vi "Control - Generic - Smoke Limit Host.vi"() -> ()   [LabVIEW 2015, in "ECS-Host.lvlib"]
uses:
  ECS-Host.lvlib
  <vilib>/addons/Software Calibration Management/XControls/TBL2D.xctl
panel:
  in  "SmokeLimitMode":bool
  in  "_Smoke Limit Mode Tab Control":enum32{"Phi", "Quantity"}(tab)
  in  "SmokeLimitPhi_Tbl":cluster{"X":sgl[], "Y":sgl[], "Z":sgl[][]}(xcontrol)
  out "SmokeLimitPhi_TblOut":sgl caption="[]"
  in  "SmokeLimitFuel_Tbl":cluster{"X":sgl[], "Y":sgl[], "Z":sgl[][]}(xcontrol)
  out "SmokeLimitFuel_TblOut":sgl caption="[mg/cyc]"
  out "FuelLimit_Calc":sgl caption="[]"
  in  "SmokeLimit_E":bool
  out "SmokeLimitActive":bool
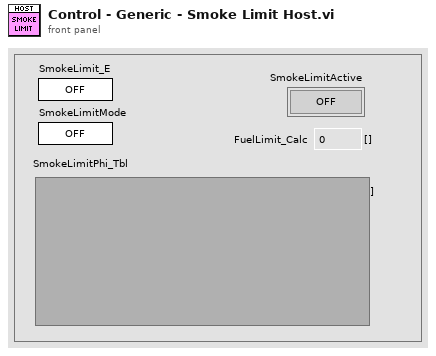
[diagram p1: front panel]
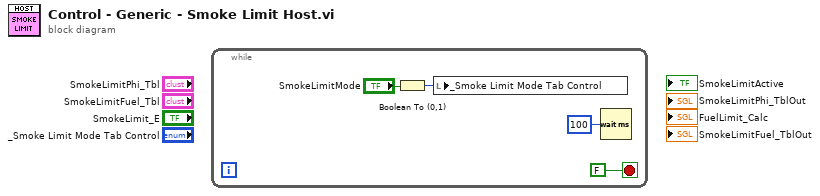
[diagram p0: block diagram]
diagram:
  n1 = while {
    stop <- FALSE stop-if-true
    n2 = Boolean To (0,1)(Boolean="SmokeLimitMode") -> (0, 1=w1:i16)
    n3 = local write "_Smoke Limit Mode Tab Control"(w1) -> ()
    n4 = Wait (ms)(milliseconds to wait=u32 100) -> ()  [unwired: 1 out]
  }
